vi "read_data0611.vi"() -> ()   [LabVIEW 2013]
uses:
  <vilib>/Utility/file.llb/Read From Spreadsheet File (DBL).vi
  <vilib>/gmath/interp.llb/Interpolate 2D Scattered (2D).vi
  <vilib>/Math Plots/3D Math Plots/3D Scatter/3D Scatter Datatype/Public/Plot Helper (Vector).vi
  <vilib>/Utility/file.llb/Write To Spreadsheet File (DBL).vi
  <vilib>/Analysis/NI_AALBase.lvlib
  <vilib>/Math Plots/3D Math Plots/3D Scatter/3D Scatter Datatype/3D Scatter Datatype.lvclass
  <vilib>/gmath/NI_AAL_Interpolation.lvlib
panel:
  out "transposed array 2":dbl[][](array[numeric])
  out "XY Graph 4":cluster{"X":dbl, "Y":dbl}[](graph)
  out "XY Graph 3":T1(graph)
  out "appended array":dbl[](array[numeric])
  out "XY Graph 2":cluster{"X":dbl, "Y":dbl}[](graph)
  out "Waveform Graph":dbl[](graph)
  out "XY Graph":cluster{"X":dbl, "Y":dbl}[](graph)
  out "transposed array":dbl[][](array[numeric])
  out "File open":path
  out "appended path 2":path
  out "filenames":string[](array[string])
  out "folder names":string[](array[string])
  out "appended path":path
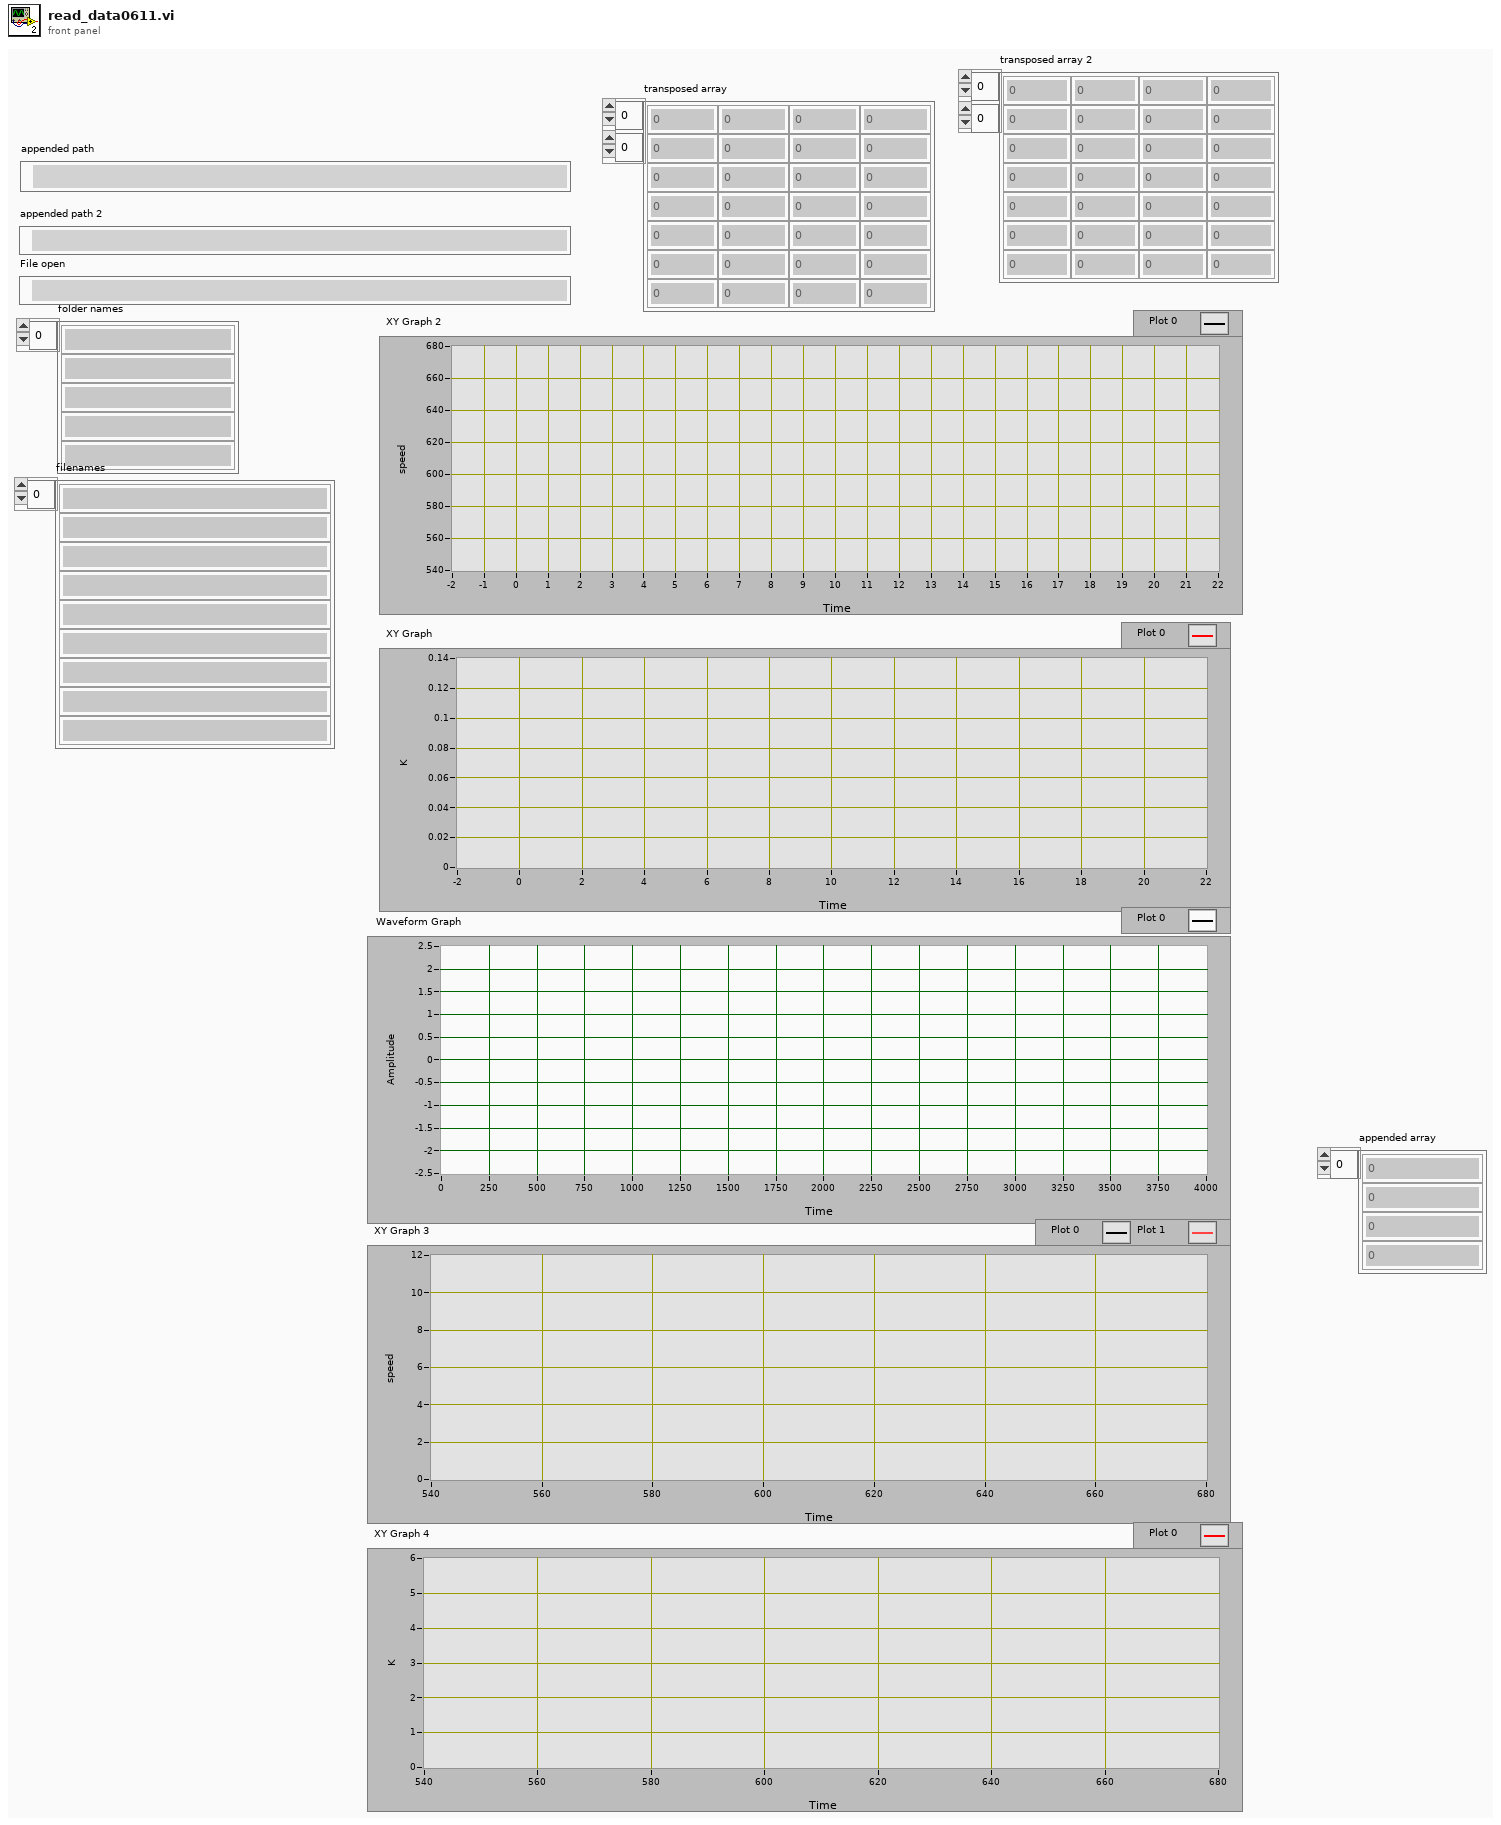
[diagram p1: front panel]
types:
  T1 = cluster{"Speed":dbl, "Torque":dbl, "Torque_O":dbl}[]
  T2 = enum16{"open", "replace", "create", "open or create", "replace or create", "replace or create with confirmation"}
  T3 = cluster{"Speed":dbl, "Torque":dbl, "K":dbl, "Air gap distance ":dbl, "Torque_O":dbl}
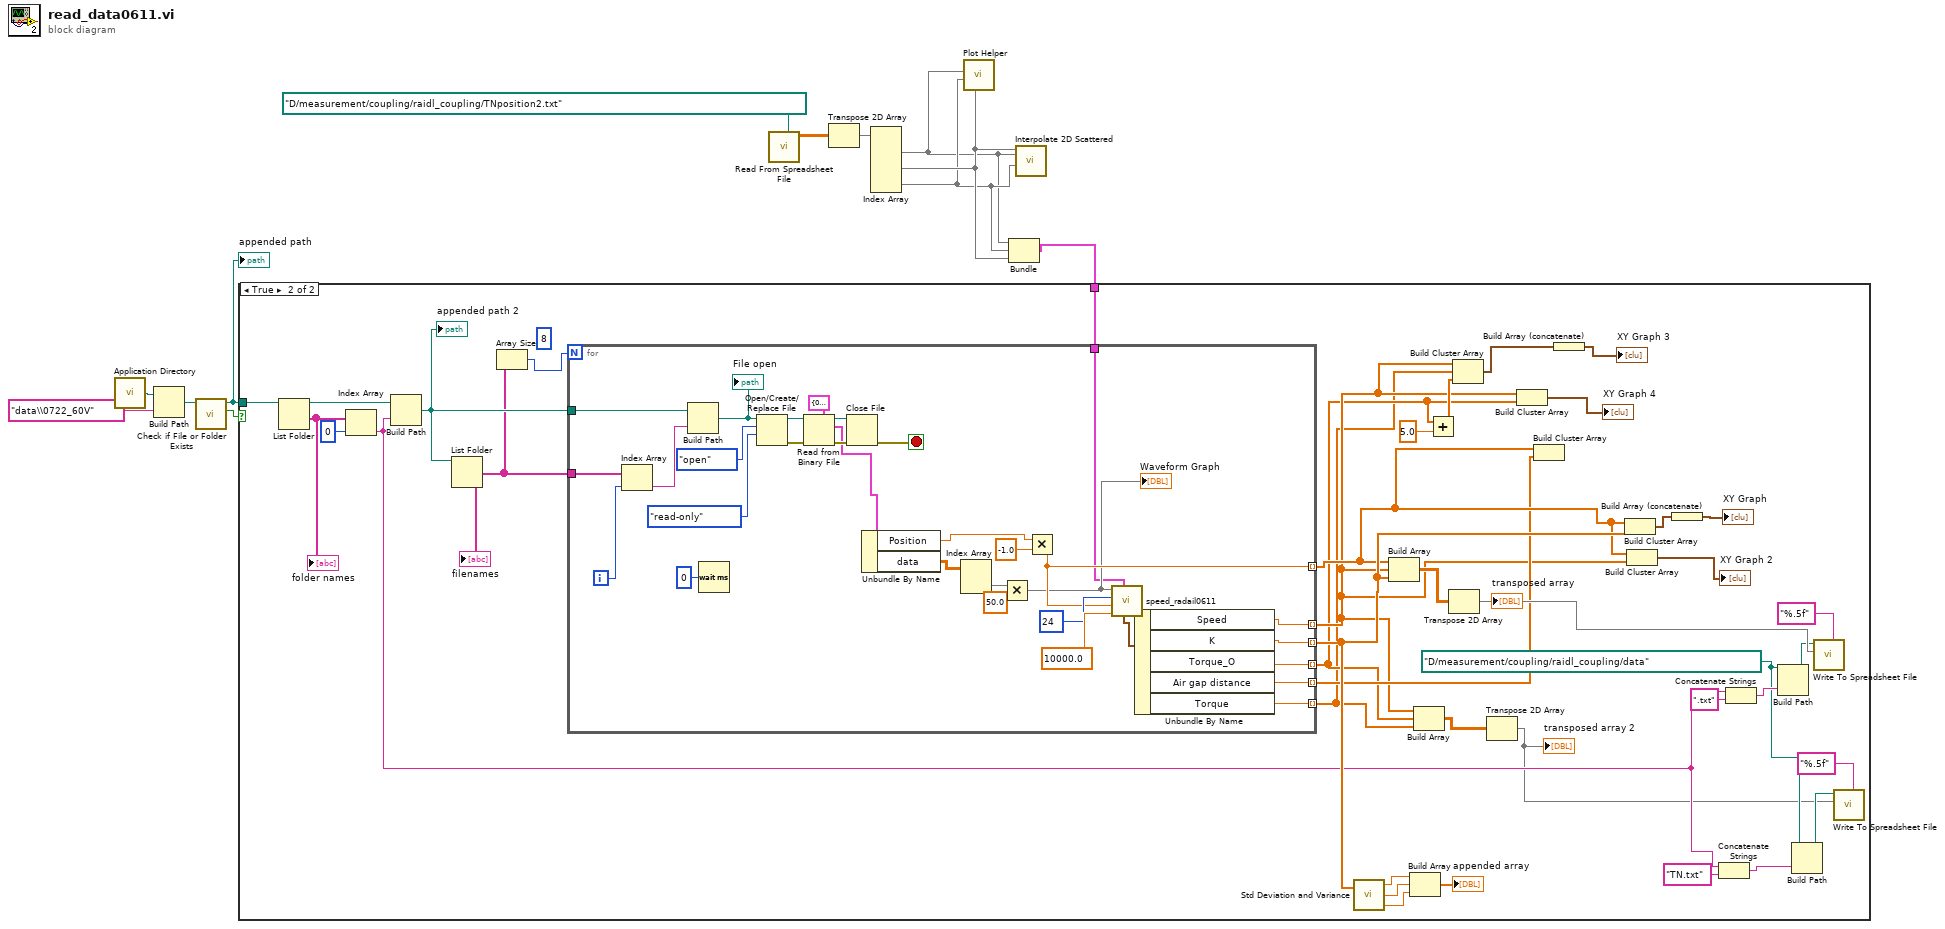
[diagram p0: block diagram]
diagram:
  n1 = call <vilib>:"Application Directory.vi"() -> ("Application Directory"=w12:path)
  n2 = Build Path(base path=w12, name or relative path="data\\0722_60V") -> (appended path=w10:path)
  n3 = call <vilib>:"Check if File or Folder Exists.vi"("path"=w10) -> ("file or folder exists?"=w9:bool, "dup path"=w8:path)  [unwired: 8 in, 1 out]
  "appended path" <- w8
  n4 = call-poly <vilib>:"Read From Spreadsheet File.vi"("file path (dialog if empty)"=path "D:/measurement/coupling/raidl_coupling/TNposition2.txt") -> ("all rows"=w3:dbl[][])  [unwired: 6 in, 4 out]
  n5 = Transpose 2D Array(2D array=w3) -> (transposed array=w4:dbl[][])
  n6 = Index Array(array=w4) -> (element #1=w5:dbl[], element #2=w7:dbl[], element #3=w6:dbl[])  [unwired: 6 in]
  n7 = call-poly <vilib>:"Plot Helper.vi"("z vector"=w7, "y vector"=w6, "x vector"=w5) -> ()  [unwired: 3 in, 6 out]
  n8 = Bundle(w5, w6, w7) -> (w1:cluster{dbl[], dbl[], dbl[]})  [unwired: 1 in]
  n9 = case shown="True" w9 {
    tunnel: w8 -> [_ w52]
    tunnel: w1 -> [_ w32]
    frame False {
    }
    frame True {
      (unwired) 8
      w18 = path "D:/measurement/coupling/raidl_coupling/data" ("file path (dialog if empty)")
      n10 = List Folder(path=w52) -> (path out=w51:path, folder names=w45:string[])  [unwired: 3 in, 2 out]
      "folder names" <- w45
      n11 = Index Array(array=w45, index=0 ("length")) -> (element=w19:string)
      n12 = Build Path(base path=w51, name or relative path=w19) -> (appended path=w49:path)
      "appended path 2" <- w49
      n13 = List Folder(path=w49) -> (filenames=w48:string[])  [unwired: 3 in, 3 out]
      "filenames" <- w48
      n14 = Array Size(array=w48) -> (size(s)=w29:i32)
      n15 = for {
        N: w29 -> [_]
        tunnel: w48 -> [w83]
        tunnel: w49 -> [w82]
        tunnel: [w61] -> w31 mode=indexing
        tunnel: [w60] -> w17 mode=indexing
        tunnel: [w59] -> w37 mode=indexing
        tunnel: w32 -> [w56]
        tunnel: [w55] -> w16 mode=indexing
        tunnel: [w54] -> w30 mode=indexing
        tunnel: [w53] -> w15 mode=indexing
        i -> [w58]
        stop <- w72 stop-if-true
        n16 = Index Array(array=w83, index=w58) -> (element=w81:string)
        n17 = Build Path(base path=w82, name or relative path=w81) -> (appended path=w80:path)
        "File open" <- w80
        n18 = Wait (ms)(milliseconds to wait=u32 0) -> ()  [unwired: 1 out]
        n19 = Open/Create/Replace File(file path (use dialog)=w80, operation (0:open)=T2."open", access (0:read/write)=enum16{"read/write", "read-only", "write-only"}."read-only") -> (refnum out=w77:refnum<file>, error out=w76:errorcluster)  [unwired: 3 in, 1 out]
        n20 = Read from Binary File(5:cluster{"Position":dbl, "data":dbl[][]} {"Position"=0.0, "data"=[]} ("output cluster"), 8:w76, 11:w77) -> (0:w73:errorcluster, 2:w70:cluster{"Position":dbl, "data":dbl[][]}, 3:w74:refnum<file>)  [unwired: 3 in, 1 out]
        n21 = Close File(refnum=w74, error in=w73) -> (error out=w72:errorcluster)  [unwired: 1 out]
        n22 = Unbundle By Name(w70) -> ("Position"=w63:dbl, "data"=w68:dbl[][])
        n23 = Index Array(array=w68) -> (element=w65:dbl[])  [unwired: 2 in]
        n24 = Multiply(x=w65, y=50.0) -> (x*y=w57:dbl[])
        "Waveform Graph" <- w57
        n25 = Multiply(x=w63, y=-1.0) -> (x*y=w61:dbl)
        n26 = call "speed_radail0611.vi"("XYZ Data"=w56, "rate"=10000.0, "Optical"=w61, "Pole Pair"=24, "Voltage"=w57) -> ("output Data"=w62:T3)  [unwired: 1 in, 4 out]
        n27 = Unbundle By Name(w62) -> ("Speed"=w60:dbl, "K"=w59:dbl, "Torque_O"=w55:dbl, "Air gap distance"=w54:dbl, "Torque"=w53:dbl)
      }
      n28 = call <vilib>:"Std Deviation and Variance.vi"("X"=w37) -> ("mean"=w36:dbl, "standard deviation"=w35:dbl, "variance"=w34:dbl)  [unwired: 1 in]
      n29 = Build Array(w31, w17, w37) -> (w47:dbl[][])
      n30 = Build Array(w36, w35, w34) -> (→"appended array":dbl[])
      n31 = Build Array(w17, w16, w15) -> (w14:dbl[][])
      n32 = Add(x=w16, y=5.0) -> (x+y=w24:dbl[])
      n33 = Transpose 2D Array(2D array=w47) -> (transposed array=w46:dbl[][])
      "transposed array" <- w46
      n34 = Build Cluster Array(w17, w15, w24) -> (w28:cluster{"Speed":dbl, "Torque":dbl, dbl}[])
      n35 = Transpose 2D Array(2D array=w14) -> (transposed array=w13:dbl[][])
      "transposed array 2" <- w13
      n36 = Build Cluster Array(w17, w16) -> (→"XY Graph 4":cluster{"Speed":dbl, "Torque_O":dbl}[])
      n37 = Build Cluster Array(w31, w30) -> ()  [unwired: 1 out]
      n38 = Build Array (concatenate)(w28) -> (→"XY Graph 3":cluster{"Speed":dbl, "Torque":dbl, dbl}[])
      n39 = Build Cluster Array(w31, w37) -> (w40:cluster{dbl, "K":dbl}[])
      n40 = Build Cluster Array(w31, w17) -> (→"XY Graph 2":cluster{dbl, "Speed":dbl}[])
      n41 = Build Array (concatenate)(w40) -> (→"XY Graph":cluster{dbl, "K":dbl}[])
      n42 = Concatenate Strings(w19, "TN.txt" ("string")) -> (w23:string)
      n43 = Concatenate Strings(w19, ".txt" ("string")) -> (w41:string)
      n44 = Build Path(base path=w18, name or relative path=w41) -> (appended path=w43:path)
      n45 = Build Path(base path=w18, name or relative path=w23) -> (appended path=w21:path)
      n46 = call-poly <vilib>:"Write To Spreadsheet File.vi"("format (%.3f)"="%.5f", "2D data"=w46, "file path (dialog if empty)"=w43) -> ()  [unwired: 5 in, 1 out]
      n47 = call-poly <vilib>:"Write To Spreadsheet File.vi"("format (%.3f)"="%.5f", "2D data"=w13, "file path (dialog if empty)"=w21) -> ()  [unwired: 5 in, 1 out]
    }
  }
  n48 = call-poly <vilib>:"Interpolate 2D Scattered.vi"("Y"=w6, "X"=w5, "Z"=w7) -> ()  [unwired: 7 in, 2 out]
